vi "SEQUENTIAL LAMP.vi"() -> ()   [LabVIEW 2015]
panel:
  in  "Stop Button":bool
  out "TIMER":i32
  out "R":bool
  out "Y":bool
  out "G":bool
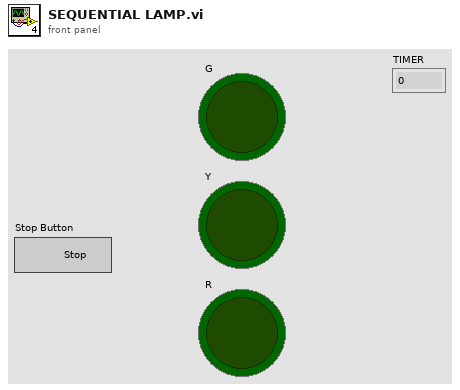
[diagram p1: front panel]
types:
  T1 = enum16{"START", "INISIALISASI", "G-ON", "Y-ON", "R-ON", "KONTINYU?", "STOP"}
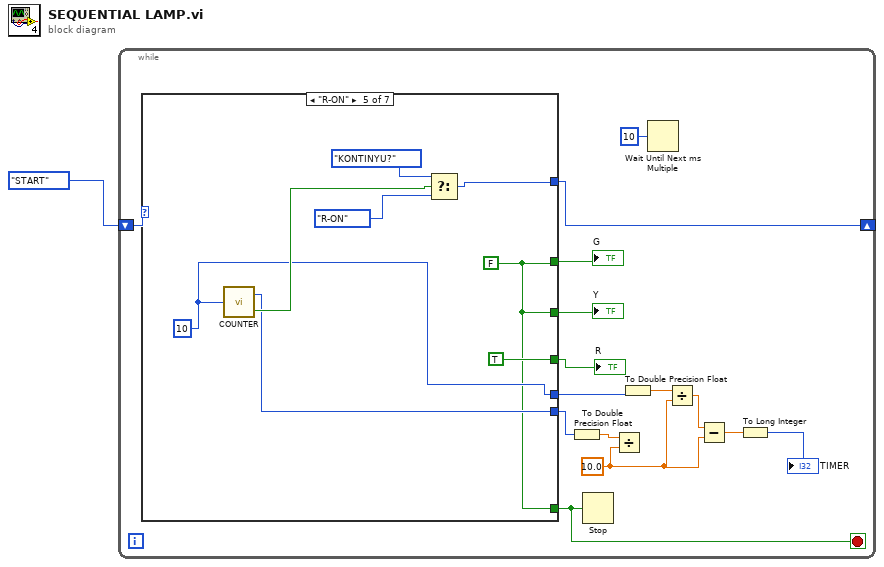
[diagram p0: block diagram]
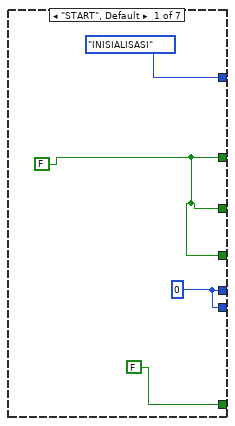
[diagram p2: hidden frame]
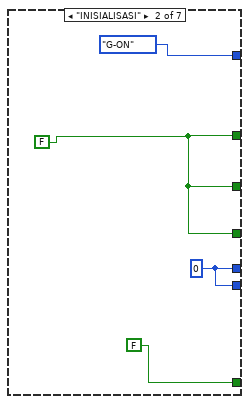
[diagram p3: hidden frame]
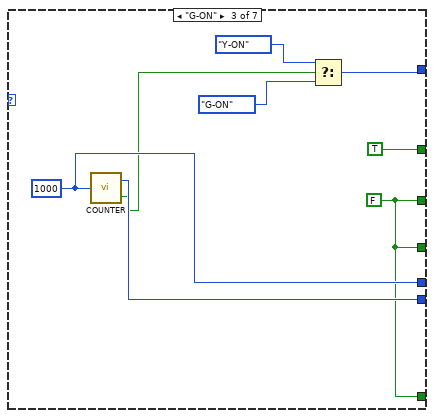
[diagram p4: hidden frame]
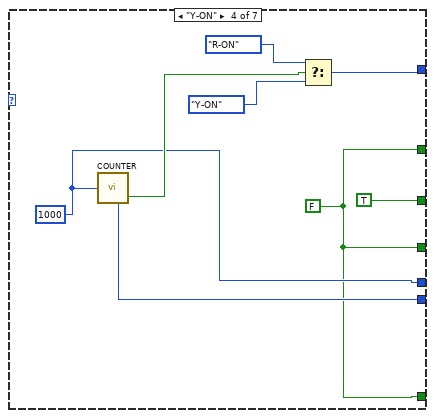
[diagram p5: hidden frame]
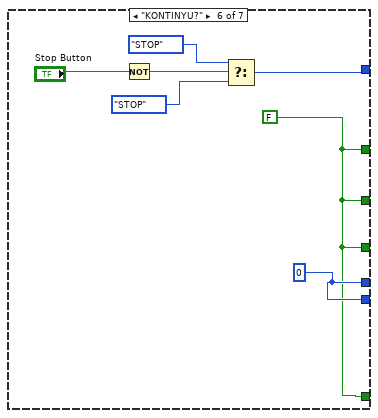
[diagram p6: hidden frame]
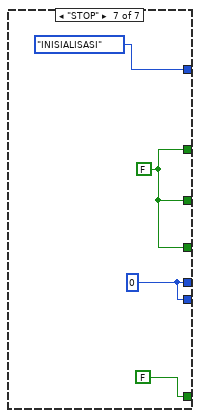
[diagram p7: hidden frame]
diagram:
  n1 = while {
    shift-right: [w15] -> _
    shift-left: T1."START" -> [w16]
    stop <- w2 stop-if-true
    w5 = 10.0 ("y")
    n2 = case shown="\"R-ON\"" w16 {
      tunnel: [T1."INISIALISASI" T1."G-ON" w27 w38 w45 w51 T1."INISIALISASI"] -> w15
      tunnel: [w19 w23 TRUE w33 w41 w50 w58] -> w14
      tunnel: [w19 w23 w26 TRUE w41 w50 w58] -> w13
      tunnel: [w19 w23 w26 w33 TRUE w50 w58] -> w12
      tunnel: [w17 w21 w31 w35 w43 w52 w56] -> w10
      tunnel: [w17 w21 w30 w34 w44 w52 w56] -> w8
      tunnel: [FALSE FALSE w26 w33 w41 w50 FALSE] -> w2
      frame "START", Default {
        w17 = 0 ("Cin")
        w19 = FALSE
      }
      frame "INISIALISASI" {
        w21 = 0 ("Cin")
        w23 = FALSE
      }
      frame "G-ON" {
        w30 = 1000 ("Cin")
        w26 = FALSE
        n3 = call "COUNTER.vi"("Cin"=w30) -> ("Cout"=w31:i32, "F"=w25:bool)
        n4 = Select(t=T1."Y-ON", s=w25, f=T1."G-ON") -> (s? t:f=w27:T1)
      }
      frame "Y-ON" {
        w34 = 1000 ("Cin")
        w33 = FALSE
        n5 = call "COUNTER.vi"("Cin"=w34) -> ("Cout"=w35:i32, "F"=w36:bool)
        n6 = Select(t=T1."R-ON", s=w36, f=T1."Y-ON") -> (s? t:f=w38:T1)
      }
      frame "R-ON" {
        w44 = 10 ("Cin")
        w41 = FALSE
        n7 = call "COUNTER.vi"("Cin"=w44) -> ("Cout"=w43:i32, "F"=w48:bool)
        n8 = Select(t=T1."KONTINYU?", s=w48, f=T1."R-ON") -> (s? t:f=w45:T1)
      }
      frame "KONTINYU?" {
        w52 = 0 ("Cin")
        w50 = FALSE
        n9 = Not(x="Stop Button") -> (.not. x?=w53:bool)
        n10 = Select(t=T1."STOP", s=w53, f=T1."STOP") -> (s? t:f=w51:T1)
      }
      frame "STOP" {
        w56 = 0 ("Cin")
        w58 = FALSE
      }
    }
    "G" <- w14
    "Y" <- w13
    "R" <- w12
    n11 = To Double Precision Float(number=w10) -> (double precision float=w9:dbl)
    n12 = Stop(stop? (T)=w2) -> ()
    n13 = Divide(x=w9, y=w5) -> ()  [unwired: 1 out]
    n14 = To Double Precision Float(number=w8) -> (double precision float=w7:dbl)
    n15 = Wait Until Next ms Multiple(millisecond multiple=u32 10) -> ()  [unwired: 1 out]
    n16 = Divide(x=w7, y=w5) -> (x/y=w6:dbl)
    n17 = Subtract(x=w6, y=w5) -> (x-y=w4:dbl)
    n18 = To Long Integer(number=w4) -> (32bit integer=→"TIMER":i32)
  }
